vi "Get Element.vi"(8 "error in (no error)":errorcluster, 10 "Key":string, 11 "SMO.Dictionary in":refnum<class "SMO.Dictionary.lvclass">) -> (0 "error out":errorcluster, 1 "Value":variant, 2 "Key dup":string, 3 "SMO.Dictionary out":refnum<class "SMO.Dictionary.lvclass">)   [LabVIEW 2013, in "SMO.Dictionary.lvlib" / "SMO.Dictionary.lvclass"]
uses:
  SMO.Dictionary.lvclass
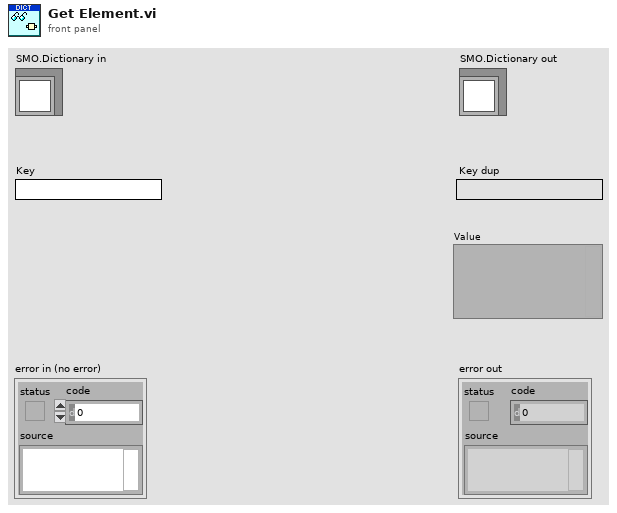
[diagram p1: front panel]
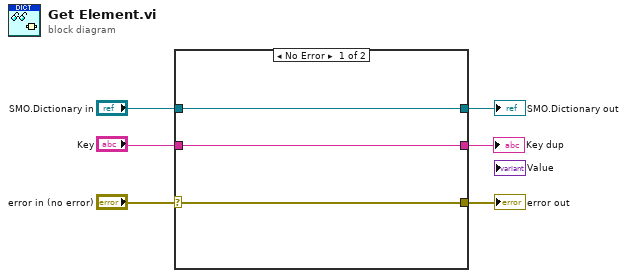
[diagram p0: block diagram]
diagram:
  n1 = case shown="No Error" "error in (no error)" {
    selector: "error in (no error)" -> [w8 w12]
    tunnel: [w8 w12] -> w5
    tunnel: [w9 w11] -> w3
    tunnel: "SMO.Dictionary in" -> [w9 w11]
    tunnel: [w7 w10] -> w2
    tunnel: "Key" -> [w7 w10]
    frame No Error {
    }
    frame Error {
    }
  }
  "error out" <- w5
  "SMO.Dictionary out" <- w3
  "Key dup" <- w2
